vi "ZeroMQ_GS.vi"() -> ()   [LabVIEW 2018]
uses:
  <vilib>/addons/zeromq/socket_type.ctl
  <vilib>/addons/zeromq/socket_options.ctl
  <vilib>/addons/zeromq/zeromq.lvlib
  <vilib>/addons/zeromq/zmq_socket.lvclass
  <vilib>/addons/zeromq/zmq_context.lvclass
panel:
  in  "stop 4":bool
  out "command 2":string
  out "error out 4":errorcluster
  out "ADDRESS SUB":string
  out "error out":errorcluster
  out "command tcpip":string
  out "response sub":string
  out "command":string
  in  "stop 3":bool
  out "error out 3":errorcluster
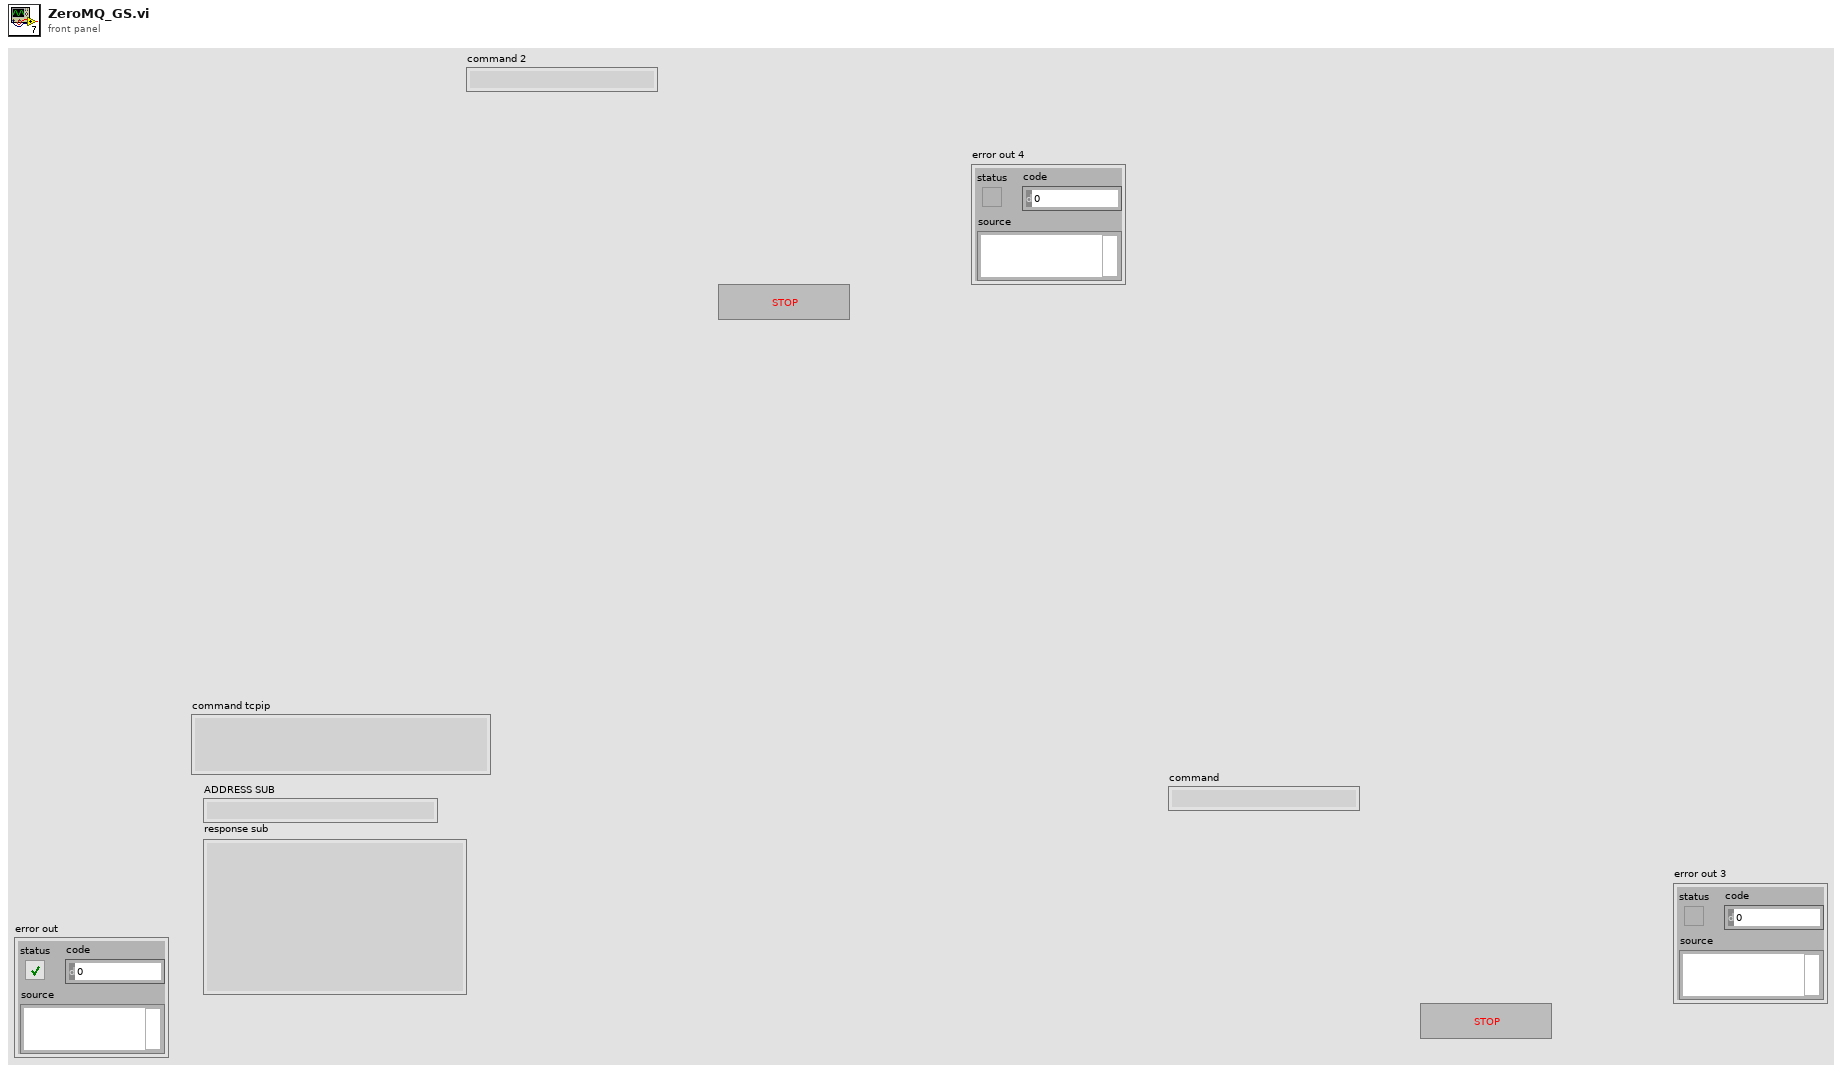
[diagram p1: front panel]
types:
  T1 = typedef "zeromq.lvlib/socket_options.ctl" = enum8{"NONE", "ZMQ_HWM", "<2>", "ZMQ_SWAP", "ZMQ_AFFINITY", "ZMQ_ROUTING_ID", "ZMQ_SUBSCRIBE", "ZMQ_UNSUBSCRIBE", "ZMQ_RATE", "ZMQ_RECOVERY_IVL", "ZMQ_MCAST_LOOP", "ZMQ_SNDBUF", "ZMQ_RCVBUF", "ZMQ_RCVMORE", "ZMQ_FD", "ZMQ_EVENTS", "ZMQ_TYPE", "ZMQ_LINGER", "ZMQ_RECONNECT_IVL", "ZMQ_BACKLOG", "ZMQ_RECOVERY_IVL_MSEC", "ZMQ_RECONNECT_IVL_MAX", "ZMQ_MAXMSGSIZE", "ZMQ_SNDHWM", "ZMQ_RCVHWM", "ZMQ_MULTICAST_HOPS", "<26>", "ZMQ_RCVTIMEO", "ZMQ_SNDTIMEO", "<29>", "<30>", "ZMQ_IPV4ONLY", "ZMQ_LAST_ENDPOINT", "ZMQ_ROUTER_MANDATORY", "ZMQ_TCP_KEEPALIVE", "ZMQ_TCP_KEEPALIVE_CNT", "ZMQ_TCP_KEEPALIVE_IDLE", "ZMQ_TCP_KEEPALIVE_INTVL", "ZMQ_TCP_ACCEPT_FILTER", "ZMQ_IMMEDIATE", "ZMQ_XPUB_VERBOSE", "ZMQ_ROUTER_RAW", "ZMQ_IPV6", "ZMQ_MECHANISM", "ZMQ_PLAIN_SERVER", "ZMQ_PLAIN_USERNAME", "ZMQ_PLAIN_PASSWORD", "ZMQ_CURVE_SERVER", "ZMQ_CURVE_PUBLICKEY", "ZMQ_CURVE_SECRETKEY", "ZMQ_CURVE_SERVERKEY", "ZMQ_PROBE_ROUTER", "ZMQ_REQ_CORRELATE", "ZMQ_REQ_RELAXED", "ZMQ_CONFLATE", "ZMQ_ZAP_DOMAIN", "ZMQ_ROUTER_HANDOVER", "ZMQ_TOS", "ZMQ_IPC_FILTER_PID", "ZMQ_IPC_FILTER_UID", "ZMQ_IPC_FILTER_GID", "ZMQ_CONNECT_ROUTING_ID", "ZMQ_GSSAPI_SERVER", "ZMQ_GSSAPI_PRINCIPAL", "ZMQ_GSSAPI_SERVICE_PRINCIPAL", "ZMQ_GSSAPI_PLAINTEXT", "ZMQ_HANDSHAKE_IVL", "<67>", "ZMQ_SOCKS_PROXY", "ZMQ_XPUB_NODROP", "ZMQ_BLOCKY", "ZMQ_XPUB_MANUAL", "ZMQ_XPUB_WELCOME_MSG", "ZMQ_STREAM_NOTIFY", "ZMQ_INVERT_MATCHING", "ZMQ_HEARTBEAT_IVL", "ZMQ_HEARTBEAT_TTL", "ZMQ_HEARTBEAT_TIMEOUT", "ZMQ_XPUB_VERBOSER", "ZMQ_CONNECT_TIMEOUT", "ZMQ_TCP_MAXRT", "ZMQ_THREAD_SAFE", "<82>", "<83>", "ZMQ_MULTICAST_MAXTPDU", "ZMQ_VMCI_BUFFER_SIZE", "ZMQ_VMCI_BUFFER_MIN_SIZE", "ZMQ_VMCI_BUFFER_MAX_SIZE", "ZMQ_VMCI_CONNECT_TIMEOUT", "ZMQ_USE_FD", "ZMQ_GSSAPI_PRINCIPAL_NAMETYPE", "ZMQ_GSSAPI_SERVICE_PRINCIPAL_NAMETYPE", "ZMQ_BINDTODEVICE", "ZMQ_ZAP_ENFORCE_DOMAIN", "ZMQ_LOOPBACK_FASTPATH", "ZMQ_METADATA", "ZMQ_MULTICAST_LOOP", "ZMQ_ROUTER_NOTIFY"}
  T2 = typedef "zeromq.lvlib/socket_type.ctl" = enum8{"ZMQ_PAIR", "ZMQ_PUB", "ZMQ_SUB", "ZMQ_REQ", "ZMQ_REP", "ZMQ_DEALER", "ZMQ_ROUTER", "ZMQ_PULL", "ZMQ_PUSH", "ZMQ_XPUB", "ZMQ_XSUB", "ZMQ_STREAM", "ZMQ_SERVER", "ZMQ_CLIENT", "ZMQ_RADIO", "ZMQ_DISH", "ZMQ_GATHER", "ZMQ_SCATTER", "ZMQ_DGRAM"}
  T3 = cluster{"ID":u32, "Address":string, "Service Name 1":string, "Service Name 2":string, "queue TX":refnum<queue>, "queue RX":refnum<queue>, "Port 1":u32, "Port 2":u32}
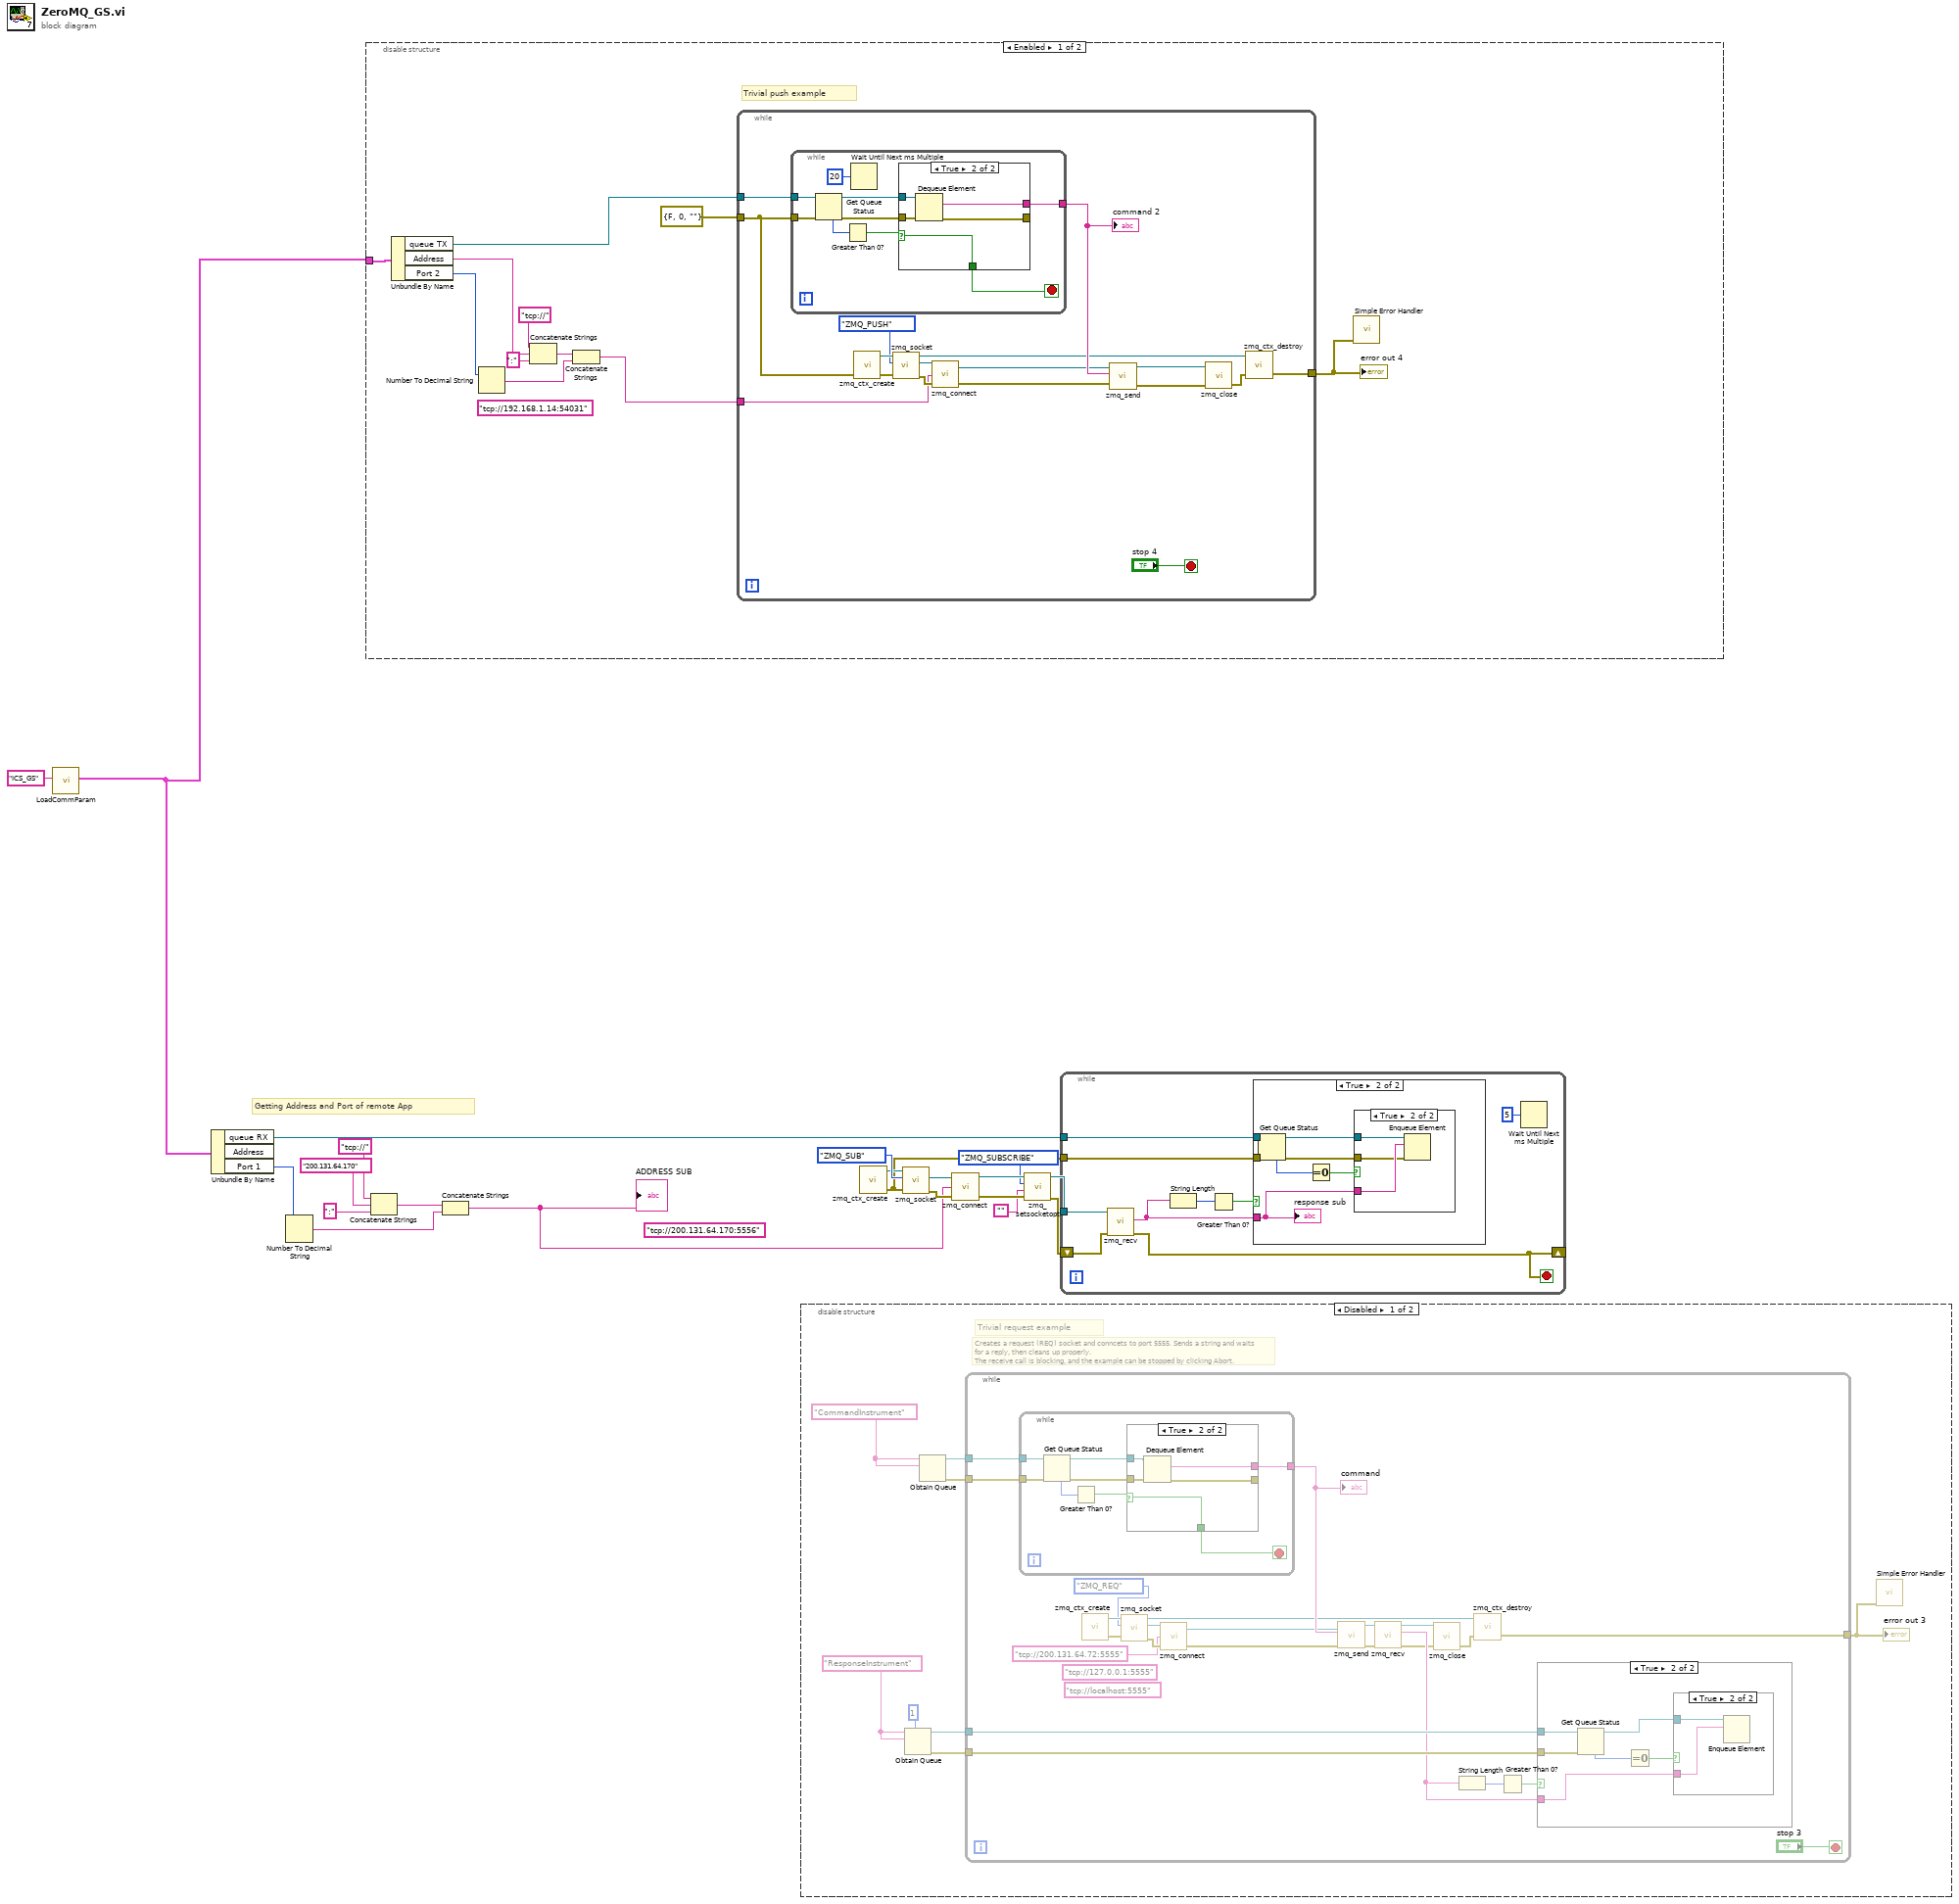
[diagram p0: block diagram]
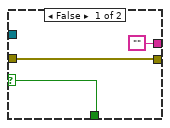
[diagram p2: hidden frame]
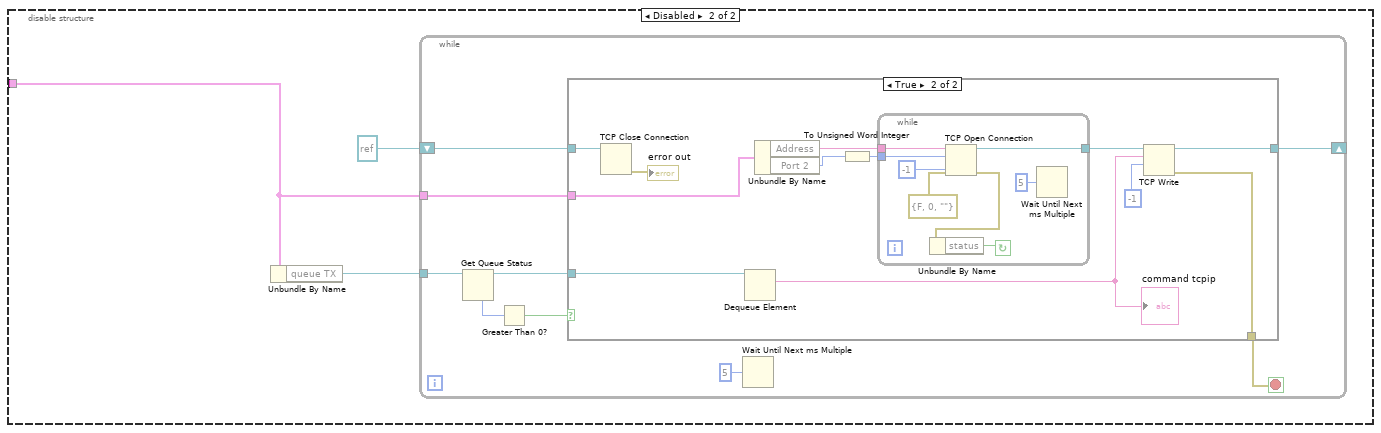
[diagram p3: hidden frame]
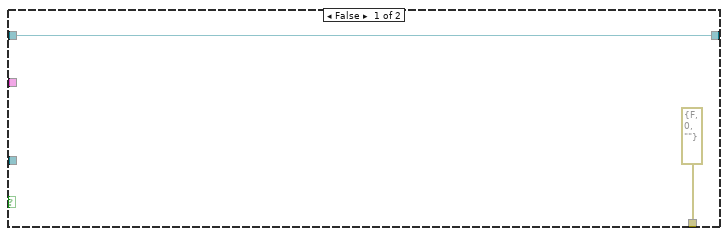
[diagram p4: hidden frame]
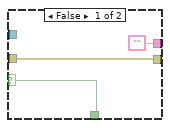
[diagram p9: hidden frame]
diagram:
  (unwired) "tcp://200.131.64.170:5556" ("endpoint")
  # "Getting Address and Port of remote App"
  n1 = call "LoadCommParam.vi"("section name"="ICS_GS") -> ("output cluster"=w1:T3)  [unwired: 10 in]
  n2 = Unbundle By Name(w1) -> ("queue RX"=w8:refnum<queue>, "Port 1"=w7:u32)  [unwired: 1 out]
  n3 = Number To Decimal String(number=w7) -> (decimal integer string=w6:string)  [unwired: 1 in]
  n4 = disable-structure shown="Enabled" {
    disable-tunnel: w1 -> [w22 w67]
    frame Enabled {
      (unwired) "tcp://192.168.1.14:54031" ("endpoint")
      # "Trivial push example"
      n5 = Unbundle By Name(w22) -> ("queue TX"=w24:refnum<queue>, "Address"=w26:string, "Port 2"=w25:u32)
      n6 = Number To Decimal String(number=w25) -> (decimal integer string=w30:string)  [unwired: 1 in]
      n7 = Concatenate Strings("tcp://" ("string"), w26, ":" ("string")) -> (w29:string)
      n8 = Concatenate Strings(w29, w30) -> (w23:string)
      n9 = while {
        tunnel: w24 -> [w49]
        tunnel: errorcluster {"status"=FALSE, "code"=0, "source"=""} ("error out") -> [w33]
        tunnel: [w38] -> w32
        tunnel: w23 -> [w34]
        stop <- "stop 4" stop-if-true
        n10 = while {
          tunnel: w49 -> [w57]
          tunnel: w33 -> [w56]
          tunnel: [w52] -> w48
          stop <- w51 stop-if-true
          n11 = Get Queue Status(queue=w57, error in (no error)=w56) -> (queue out=w53:refnum<queue>, error out=w54:errorcluster, # elements in queue=w58:i32)  [unwired: 1 in, 5 out]
          n12 = Greater Than 0?(x=w58) -> (x > 0?=w55:bool)
          n13 = Wait Until Next ms Multiple(millisecond multiple=u32 20) -> ()  [unwired: 1 out]
          n14 = case shown="True" w55 {
            selector: w55 -> [w59 w62]
            tunnel: w54 -> [w61 w66]
            tunnel: w53 -> [_ w65]
            tunnel: [w61 w64] -> _
            tunnel: ["" w63] -> w52
            tunnel: [w59 w62] -> w51
            frame False {
            }
            frame True {
              n15 = Dequeue Element(queue=w65, error in (no error)=w66) -> (element=w63:string, error out=w64:errorcluster)  [unwired: 1 in, 2 out]
            }
          }
        }
        "command 2" <- w48
        n16 = call <vilib>:"zmq_ctx_create.vi"("error in"=w33) -> ("error out"=w43:errorcluster, "context out"=w46:refnum<class "zmq_context.lvclass">)  [unwired: 3 in]
        n17 = call <vilib>:"zmq_socket.vi"("error in"=w43, "socket type"=socket_type."ZMQ_PUSH", "context in"=w46) -> ("error out"=w45:errorcluster, "socket out"=w44:refnum<class "zmq_socket.lvclass">, "context out"=w37:refnum<class "zmq_context.lvclass">)  [unwired: 2 in]
        n18 = call <vilib>:"zmq_connect.vi"("error in"=w45, "endpoint"=w34, "socket in"=w44) -> ("error out"=w40:errorcluster, "socket out"=w41:refnum<class "zmq_socket.lvclass">)  [unwired: 1 in]
        n19 = call <vilib>:"zmq_send.vi"("error in"=w40, "data"=w48, "socket in"=w41) -> ("error out"=w35:errorcluster, "socket out"=w36:refnum<class "zmq_socket.lvclass">)  [unwired: 4 in]
        n20 = call <vilib>:"zmq_close.vi"("error in"=w35, "socket"=w36) -> ("error out"=w39:errorcluster)  [unwired: 3 in]
        n21 = call <vilib>:"zmq_ctx_destroy.vi"("error in"=w39, "context in"=w37) -> ("error out"=w38:errorcluster)  [unwired: 3 in]
      }
      "error out 4" <- w32
      n22 = call <vilib>:"Simple Error Handler.vi"("error in (no error)"=w32) -> ()  [unwired: 4 in, 5 out]
    }
    frame Disabled {
      n23 = Unbundle By Name(w67) -> ("queue TX"=w69:refnum<queue>)
      n24 = while {
        tunnel: w69 -> [w78]
        tunnel: w67 -> [w73]
        shift-right: [w71] -> _
        shift-left: refnum<k5> refnum ("connection ID") -> [w70]
        stop <- w72 stop-if-true
        n25 = Get Queue Status(queue=w78) -> (queue out=w75:refnum<queue>, # elements in queue=w77:i32)  [unwired: 2 in, 6 out]
        n26 = Greater Than 0?(x=w77) -> (x > 0?=w76:bool)
        n27 = case shown="True" w76 {
          tunnel: w75 -> [_ w92]
          tunnel: w73 -> [_ w90]
          tunnel: [errorcluster {"status"=FALSE, "code"=0, "source"=""} ("error out") w84] -> w72
          tunnel: [w79 w83] -> w71
          tunnel: w70 -> [w79 w81]
          frame False {
          }
          frame True {
            n28 = TCP Close Connection(connection ID=w81) -> (error out=→"error out":errorcluster)  [unwired: 2 in, 1 out]
            n29 = Dequeue Element(queue=w92) -> (element=w91:string)  [unwired: 2 in, 3 out]
            "command tcpip" <- w91
            n30 = Unbundle By Name(w90) -> ("Address"=w86:string, "Port 2"=w85:u32)
            n31 = To Unsigned Word Integer(number=w85) -> (unsigned 16bit integer=w87:u16)
            n32 = while {
              tunnel: [w100] -> w89
              tunnel: w87 -> [w99]
              tunnel: w86 -> [w98]
              stop <- w94 continue-if-true
              n33 = TCP Open Connection(address=w98, remote port or service name=w99, timeout ms (60000)=-1, error in (no error)=errorcluster {"status"=FALSE, "code"=0, "source"=""}) -> (connection ID=w100:refnum<k5>, error out=w95:errorcluster)  [unwired: 1 in]
              n34 = Unbundle By Name(w95) -> ("status"=w94:bool)
              n35 = Wait Until Next ms Multiple(millisecond multiple=u32 5) -> ()  [unwired: 1 out]
            }
            n36 = TCP Write(connection ID=w89, data in=w91, 9:-1 ("timeout ms (25000)")) -> (connection ID out=w83:refnum<k5>, error out=w84:errorcluster)  [unwired: 1 in, 1 out]
          }
        }
        n37 = Wait Until Next ms Multiple(millisecond multiple=u32 5) -> ()  [unwired: 1 out]
      }
    }
  }
  n38 = Concatenate Strings("tcp://" ("string"), "200.131.64.170" ("string"), ":" ("string")) -> (w5:string)
  n39 = Concatenate Strings(w5, w6) -> (w10:string)
  "ADDRESS SUB" <- w10
  n40 = disable-structure shown="Disabled" {
    frame Disabled {
      w101 = "ResponseInstrument"
      w102 = "CommandInstrument"
      # "Creates a request (REQ) socket and conncets to port 5555. Sends a string and waits for a reply, then cleans up properly.\nThe receive call is blocking, and the example can be stopped by clicking Abort."
      # "Trivial request example"
      n41 = Obtain Queue(max queue size (-1, unlimited)=1, name (unnamed)=w101, element data type=w101) -> (queue out=w105:refnum<queue>, error out=w104:errorcluster)  [unwired: 2 in, 1 out]
      n42 = Obtain Queue(name (unnamed)=w102, element data type=w102) -> (queue out=w107:refnum<queue>, error out=w106:errorcluster)  [unwired: 3 in, 1 out]
      n43 = while {
        tunnel: w107 -> [w130]
        tunnel: w106 -> [w129]
        tunnel: w105 -> [w127]
        tunnel: w104 -> [w126]
        tunnel: [w113] -> w103
        stop <- "stop 3" stop-if-true
        (unwired) "tcp://127.0.0.1:5555" ("endpoint")
        (unwired) "tcp://localhost:5555" ("endpoint")
        n44 = while {
          tunnel: w130 -> [w147]
          tunnel: w129 -> [w146]
          tunnel: [w142] -> w128
          stop <- w141 stop-if-true
          n45 = Get Queue Status(queue=w147, error in (no error)=w146) -> (queue out=w143:refnum<queue>, error out=w144:errorcluster, # elements in queue=w148:i32)  [unwired: 1 in, 5 out]
          n46 = Greater Than 0?(x=w148) -> (x > 0?=w145:bool)
          n47 = case shown="True" w145 {
            selector: w145 -> [w149 w152]
            tunnel: w144 -> [w151 w156]
            tunnel: w143 -> [_ w155]
            tunnel: [w151 w154] -> _
            tunnel: ["" w153] -> w142
            tunnel: [w149 w152] -> w141
            frame False {
            }
            frame True {
              n48 = Dequeue Element(queue=w155, error in (no error)=w156) -> (element=w153:string, error out=w154:errorcluster)  [unwired: 1 in, 2 out]
            }
          }
        }
        "command" <- w128
        n49 = call <vilib>:"zmq_ctx_create.vi"() -> ("error out"=w118:errorcluster, "context out"=w121:refnum<class "zmq_context.lvclass">)  [unwired: 4 in]
        n50 = call <vilib>:"zmq_socket.vi"("error in"=w118, "socket type"=socket_type."ZMQ_REQ", "context in"=w121) -> ("error out"=w120:errorcluster, "socket out"=w119:refnum<class "zmq_socket.lvclass">, "context out"=w110:refnum<class "zmq_context.lvclass">)  [unwired: 2 in]
        n51 = call <vilib>:"zmq_connect.vi"("error in"=w120, "endpoint"="tcp://200.131.64.72:5555", "socket in"=w119) -> ("error out"=w115:errorcluster, "socket out"=w116:refnum<class "zmq_socket.lvclass">)  [unwired: 1 in]
        n52 = call <vilib>:"zmq_send.vi"("error in"=w115, "data"=w128, "socket in"=w116) -> ("error out"=w131:errorcluster, "socket out"=w132:refnum<class "zmq_socket.lvclass">)  [unwired: 4 in]
        n53 = call <vilib>:"zmq_recv.vi"("error in"=w131, "socket in"=w132) -> ("error out"=w112:errorcluster, "data"=w124:string, "socket out"=w111:refnum<class "zmq_socket.lvclass">)  [unwired: 3 in, 2 out]
        n54 = call <vilib>:"zmq_close.vi"("error in"=w112, "socket"=w111) -> ("error out"=w114:errorcluster)  [unwired: 3 in]
        n55 = String Length(string=w124) -> (length=w125:i32)
        n56 = call <vilib>:"zmq_ctx_destroy.vi"("error in"=w114, "context in"=w110) -> ("error out"=w113:errorcluster)  [unwired: 3 in]
        n57 = Greater Than 0?(x=w125) -> (x > 0?=w123:bool)
        n58 = case shown="True" w123 {
          tunnel: w127 -> [_ w137]
          tunnel: w124 -> [_ w134]
          tunnel: w126 -> [_ w133]
          frame False {
          }
          frame True {
            n59 = Get Queue Status(queue=w137, error in (no error)=w133) -> (queue out=w135:refnum<queue>, # elements in queue=w138:i32)  [unwired: 1 in, 6 out]
            n60 = Equal To 0?(x=w138) -> (x = 0?=w136:bool)
            n61 = case shown="True" w136 {
              tunnel: w135 -> [_ w140]
              tunnel: w134 -> [_ w139]
              frame False {
              }
              frame True {
                n62 = Enqueue Element(queue=w140, element=w139) -> ()  [unwired: 2 in, 3 out]
              }
            }
          }
        }
      }
      "error out 3" <- w103
      n63 = call <vilib>:"Simple Error Handler.vi"("error in (no error)"=w103) -> ()  [unwired: 4 in, 5 out]
    }
    frame Enabled {
    }
  }
  n64 = call <vilib>:"zmq_ctx_create.vi"() -> ("error out"=w9:errorcluster, "context out"=w11:refnum<class "zmq_context.lvclass">)  [unwired: 4 in]
  n65 = call <vilib>:"zmq_socket.vi"("error in"=w9, "socket type"=socket_type."ZMQ_SUB", "context in"=w11) -> ("error out"=w19:errorcluster, "socket out"=w12:refnum<class "zmq_socket.lvclass">)  [unwired: 2 in, 1 out]
  n66 = call <vilib>:"zmq_connect.vi"("error in"=w19, "endpoint"=w10, "socket in"=w12) -> ("error out"=w17:errorcluster, "socket out"=w18:refnum<class "zmq_socket.lvclass">)  [unwired: 1 in]
  n67 = call <vilib>:"zmq_setsocketopt.vi"("error in"=w17, "value"="", "option"=socket_options."ZMQ_SUBSCRIBE", "socket in"=w18) -> ("error out"=w16:errorcluster, "socket out"=w15:refnum<class "zmq_socket.lvclass">)  [unwired: 2 in]
  n68 = while {
    tunnel: w15 -> [w158]
    tunnel: w8 -> [w161]
    shift-right: [w164] -> _
    shift-left: w16 -> [w165]
    tunnel: w9 -> [w159]
    stop <- w164 stop-if-true
    n69 = call <vilib>:"zmq_recv.vi"("error in"=w165, "socket in"=w158) -> ("error out"=w164:errorcluster, "data"=w160:string)  [unwired: 3 in, 3 out]
    n70 = String Length(string=w160) -> (length=w163:i32)
    n71 = Greater Than 0?(x=w163) -> (x > 0?=w162:bool)
    n72 = case shown="True" w162 {
      tunnel: w161 -> [_ w171]
      tunnel: w160 -> [_ w168]
      tunnel: w159 -> [_ w167]
      frame False {
      }
      frame True {
        n73 = Get Queue Status(queue=w171, error in (no error)=w167) -> (queue out=w169:refnum<queue>, error out=w166:errorcluster, # elements in queue=w172:i32)  [unwired: 1 in, 5 out]
        n74 = Equal To 0?(x=w172) -> (x = 0?=w170:bool)
        n75 = case shown="True" w170 {
          tunnel: w169 -> [_ w175]
          tunnel: w168 -> [_ w174]
          tunnel: w166 -> [_ w173]
          frame False {
          }
          frame True {
            n76 = Enqueue Element(queue=w175, element=w174, error in (no error)=w173) -> ()  [unwired: 1 in, 3 out]
          }
        }
        "response sub" <- w168
      }
    }
    n77 = Wait Until Next ms Multiple(millisecond multiple=u32 5) -> ()  [unwired: 1 out]
  }
